vi "Subscribe to Filing Modules.vi"(8 "error in (no error)":errorcluster, 11 "Log Record in":refnum<class "Log Record.lvclass">) -> (0 "error out":errorcluster, 3 "Log Record out":refnum<class "Log Record.lvclass">)   [LabVIEW 2020, in "Log Record.lvclass"]
uses:
  Log Record.lvclass
  Log Record.lvclass/Log Record.ctl
  Template Module Messages/Subscribe Request Msg/Subscribe Request Msg.lvclass
  <vilib>/ActorFramework/Actor/Actor.lvclass
  C:/GitHub/LabActor/Process Object/Process Object.lvclass
  C:/GitHub/LabActor/Worker/Worker.lvclass
  C:/GitHub/LabActor/Template Module/Template Module.lvclass
  C:/Program Files/National Instruments/LabVIEW 2020/vi.lib/ActorFramework/Actor/Actor.lvclass
  C:/GitHub/LabActor/Post-Processors/Log Record/Log Record.lvclass
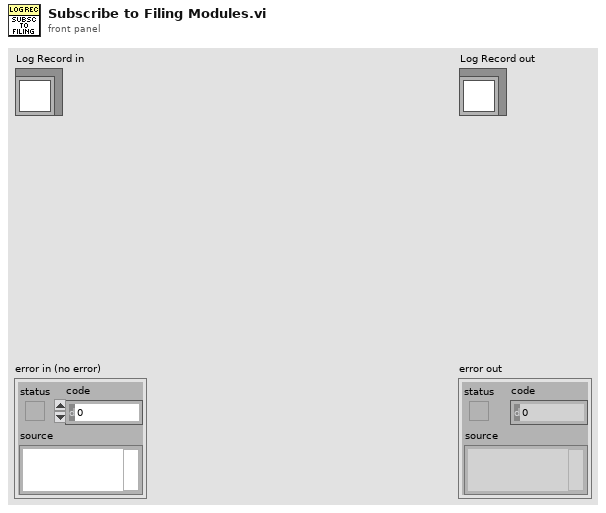
[diagram p1: front panel]
types:
  T1 = typedef "Log Record Configuration.ctl" = cluster{"OSF node  ID":string, "Conection timeout":dbl, "Station":string, "Log server ":string, "Upload to OSF":bool, "Append to lab book":bool, "Filing moduled":string[]}
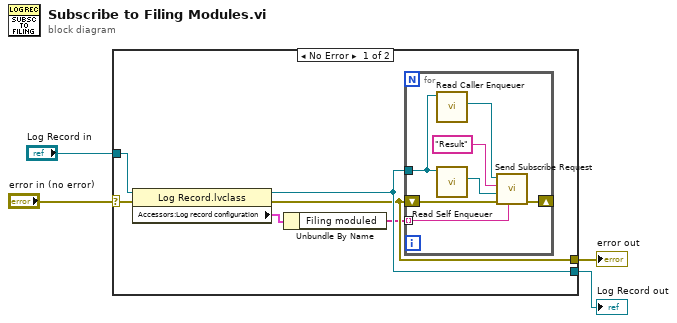
[diagram p0: block diagram]
diagram:
  n1 = case shown="No Error" "error in (no error)" {
    selector: "error in (no error)" -> [w10 w19]
    tunnel: [w7 w19] -> w3
    tunnel: [w8 w18] -> w1
    tunnel: "Log Record in" -> [w9 w18]
    frame No Error {
      n2 = property class="Log Record.lvclass"(reference=w9, error in=w10) -> (reference out=w8:refnum<class "Log Record.lvclass">, error out=w7:errorcluster, "Accessors:Log record configuration"=w6:T1)
      n3 = Unbundle By Name(w6) -> ("Filing moduled"=w5:string[])
      n4 = for {
        tunnel: w8 -> [w17]
        shift-right: [w15] -> _
        shift-left: w7 -> [w16]
        tunnel: w5 -> [w14] mode=indexing
        n5 = call <vilib>:"Read Caller Enqueuer.vi"("Actor"=w17) -> ("Caller Enqueuer"=w12:refnum<class "Message Enqueuer.lvclass">)  [unwired: 10 in]
        n6 = call <vilib>:"Read Self Enqueuer.vi"("Actor"=w17) -> ("Self Enqueuer"=w13:refnum<class "Message Enqueuer.lvclass">)  [unwired: 10 in]
        n7 = call "Send Subscribe Request.vi"("Broadcaster"=w14, "error in (no error)"=w16, "Subscriber Enqueuer"=w13, "Topic"="Result", "Message Enqueuer"=w12) -> ("error out"=w15:errorcluster)  [unwired: 5 in, 1 out]
      }
    }
    frame Error {
    }
  }
  "error out" <- w3
  "Log Record out" <- w1
